vi "CreateQuickNoteFile.vi"(8 "error in (no error)":errorcluster, 9 "String":string, 10 "created path":path, 11 "GRMActor in":refnum<class "DataLoggerUI.lvclass">) -> (0 "error out":errorcluster, 1 "String dup":string, 2 "created path dup":path, 3 "GRMActor out":refnum<class "DataLoggerUI.lvclass">)   [LabVIEW 2020, in "DataLoggerUI.lvlib" / "DataLoggerUI.lvclass"]
uses:
  DataLoggerUI/DataLoggerUI.lvclass
  DataLoggerUI/DataLoggerUI.lvclass/DataLoggerUI.ctl
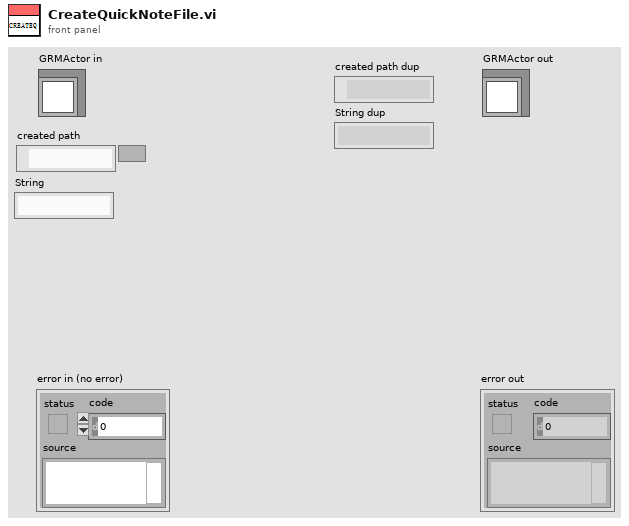
[diagram p1: front panel]
types:
  T1 = enum16{"open", "replace", "create", "open or create", "replace or create", "replace or create with confirmation"}
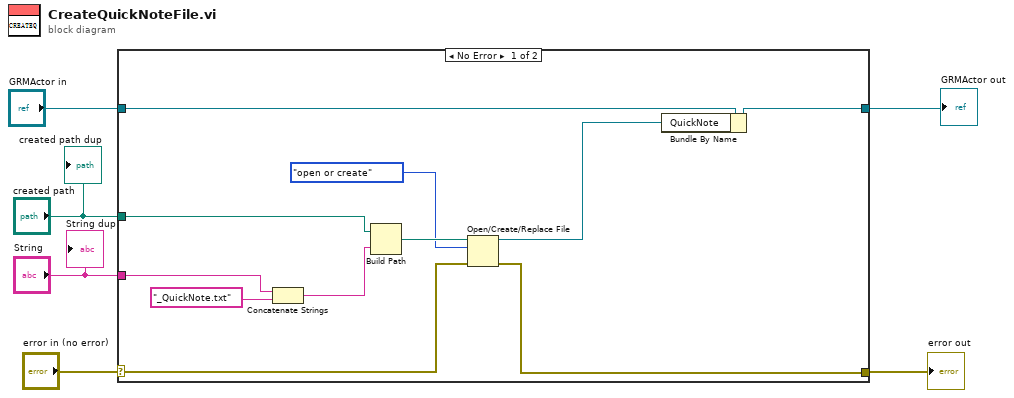
[diagram p0: block diagram]
diagram:
  n1 = case shown="No Error" "error in (no error)" {
    selector: "error in (no error)" -> [w12 w19]
    tunnel: [w10 w19] -> w5
    tunnel: [w8 w18] -> w1
    tunnel: "GRMActor in" -> [w9 w18]
    tunnel: "created path" -> [w14 _]
    tunnel: "String" -> [w16 _]
    frame No Error {
      n2 = Concatenate Strings(w16, "_QuickNote.txt" ("string")) -> (w15:string)
      n3 = Build Path(base path=w14, name or relative path=w15) -> (appended path=w13:path)
      n4 = Open/Create/Replace File(file path (use dialog)=w13, error in=w12, operation (0:open)=T1."open or create") -> (refnum out=w7:refnum<file>, error out=w10:errorcluster)  [unwired: 3 in, 1 out]
      n5 = Bundle By Name(cluster=w9, "QuickNote"=w7) -> (w8:refnum<class "DataLoggerUI.lvclass">)
    }
    frame Error {
    }
  }
  "error out" <- w5
  "GRMActor out" <- w1
  "created path dup" <- "created path"
  "String dup" <- "String"
